vi "Set As Main VI Core.vi"(8 "error in (no error)":errorcluster, 11 "Calling VI Ref in":refnum<vi>) -> (0 "error out":errorcluster, 3 "Calling VI Ref out":refnum<vi>)   [LabVIEW 2016]
uses:
  <userlib>/_OpenG.lib/file/file.llb/Compare Two Paths - Scalar__ogtk.vi
  <vilib>/Utility/error.llb/Error Cluster From Error Code.vi
  <vilib>/regexp/Match Regular Expression.xnode
  <vilib>/ErrorRing/Error Ring.xnode
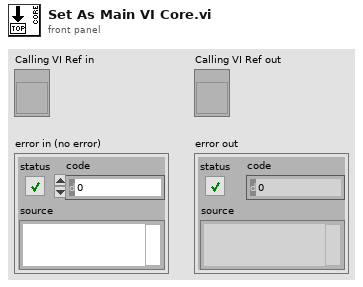
[diagram p1: front panel]
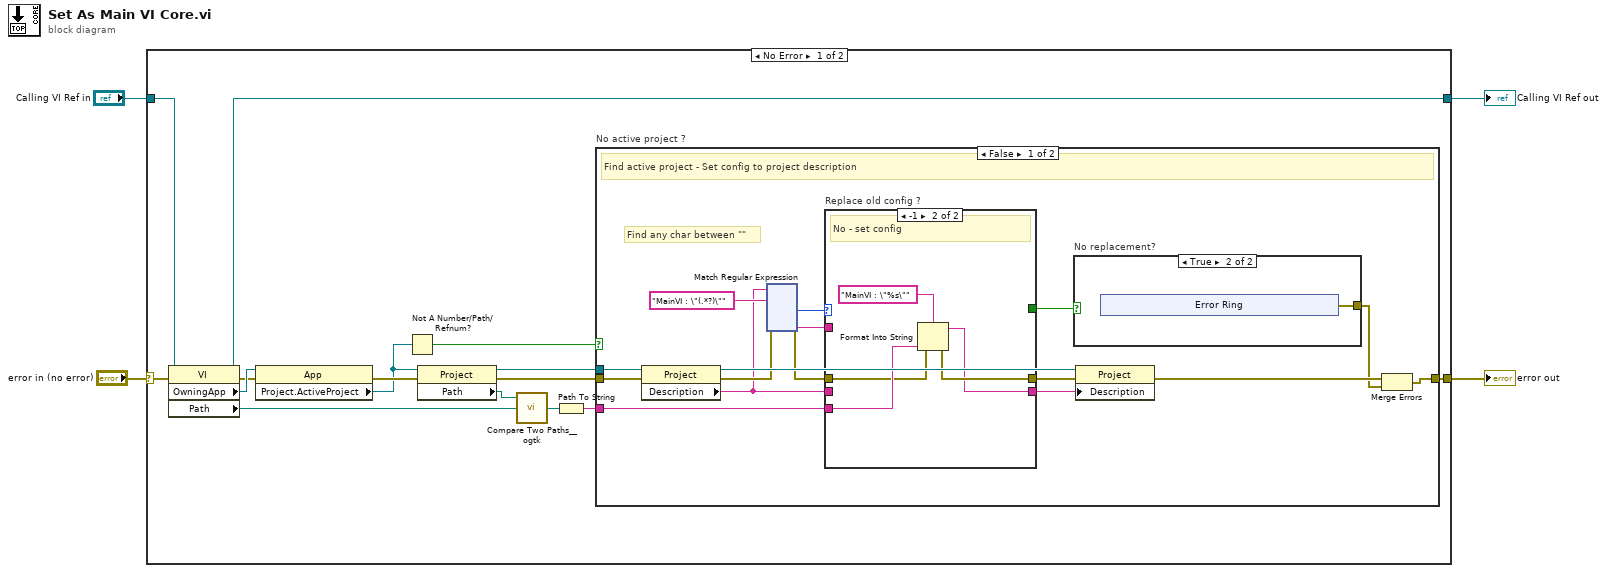
[diagram p0: block diagram]
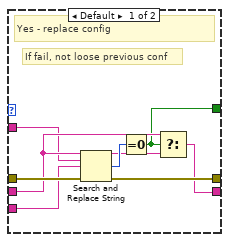
[diagram p3: hidden frame]
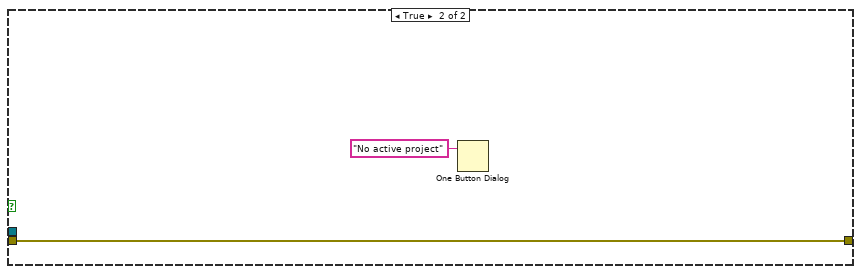
[diagram p4: hidden frame]
diagram:
  n1 = case shown="No Error" "error in (no error)" {
    selector: "error in (no error)" -> [w16 w175]
    tunnel: [w14 w175] -> w3
    tunnel: "Calling VI Ref in" -> [w15 w174]
    tunnel: [w13 w174] -> w1
    frame No Error {
      n2 = property class="VI"(reference=w15, error in=w16) -> (reference out=w13:refnum<vi>, error out=w18:errorcluster, "OwningApp"=w19:refnum<vi>, "Path"=w6:path)
      n3 = property class="App"(reference=w19, error in=w18) -> (error out=w11:errorcluster, "Project.ActiveProject"=w8:refnum<vi>)  [unwired: 1 out]
      n4 = Not A Number/Path/Refnum?(number/path/refnum=w8) -> (NaN/Path/Refnum?=w17:bool)
      n5 = property class="Project"(reference=w8, error in=w11) -> (reference out=w9:refnum<vi>, error out=w10:errorcluster, "Path"=w7:path)
      n6 = call-poly <userlib>:"Compare Two Paths__ogtk.vi"("path2"=w6, "path1"=w7) -> ("relative path from 1 to 2"=w5:path)  [unwired: 1 in, 2 out]
      n7 = Path To String(path=w5) -> (string=w12:string)
      n8 = case "No active project ?" shown="False" w17 {
        tunnel: w10 -> [w33 w172]
        tunnel: [w22 w172] -> w14
        tunnel: w9 -> [w32 _]
        tunnel: w12 -> [w27 _]
        frame False {
          # "Find any char between \"\""
          # "Find active project - Set config to project description"
          n9 = property class="Project"(reference=w32, error in=w33) -> (reference out=w31:refnum<vi>, error out=w30:errorcluster, "Description"=w26:string)
          n10 = xnode "Match Regular Expression"("input string"=w26, "regular expression"="MainVI : \"(.*?)\"", "error in"=w30) -> ("offset past match"=w21:i32, "error out"=w29:errorcluster, "submatch 1"=w20:string)  [unwired: 3 in, 3 out]
          n11 = case "Replace old config ?" shown="-1" w21 {
            tunnel: [w165 w171] -> w35
            tunnel: w27 -> [w164 w169]
            tunnel: [w162 w168] -> w34
            tunnel: w29 -> [w166 w167]
            tunnel: w26 -> [w161 _]
            tunnel: [w159 _] -> w25
            tunnel: w20 -> [w158 _]
            frame Default {
              # "If fail, not loose previous conf"
              # "Yes - replace config"
              n12 = Search and Replace String(input string=w161, search string=w158, replace string=w164, error in=w166) -> (result string=w160:string, number of replacements=w163:i32, error out=w165:errorcluster)  [unwired: 4 in, 1 out]
              n13 = Equal To 0?(x=w163) -> (x = 0?=w159:bool)
              n14 = Select(t=w161, s=w159, f=w160) -> (s? t:f=w162:string)
            }
            frame -1 {
              # "No - set config"
              n15 = Format Into String(format string="MainVI : \"%s\"" ("regular expression"), error in=w167, w169) -> (resulting string=w168:string, error out=w171:errorcluster)  [unwired: 1 in]
            }
          }
          n16 = case "No replacement?" shown="True" w25 {
            tunnel: [_ w152] -> w23
            frame False {
            }
            frame True {
              n17 = xnode "Error Ring"() -> ("error out"=w152:errorcluster)
            }
          }
          n18 = property class="Project"(reference=w31, error in=w35, "Description"=w34) -> (error out=w24:errorcluster)  [unwired: 1 out]
          n19 = Merge Errors(w24, w23) -> (w22:errorcluster)
        }
        frame True {
          n20 = One Button Dialog(message="No active project") -> ()  [unwired: 1 in, 1 out]
        }
      }
    }
    frame Error {
    }
  }
  "error out" <- w3
  "Calling VI Ref out" <- w1
